vi "_037.vi"() -> ()   [LabVIEW 2024]
panel:
  out "C":dbl
  in  "B":dbl
  in  "A":dbl
  in  "Ring":u16(ring) items=["Add"=10, "Sub"=20, "Mul"=30, "Div"=40]
  out "C":dbl
  in  "B":dbl
  in  "A":dbl
  in  "Enum":enum16{"Add", "Sub", "Mul", "Div"}(ring)
  # "Enum :"
  # "Ring :"
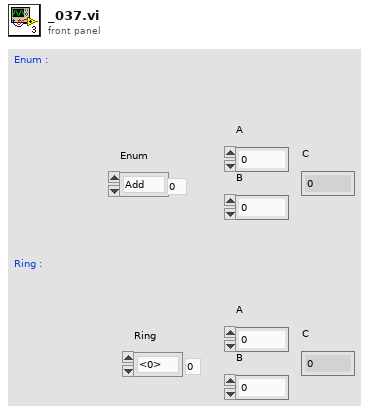
[diagram p1: front panel]
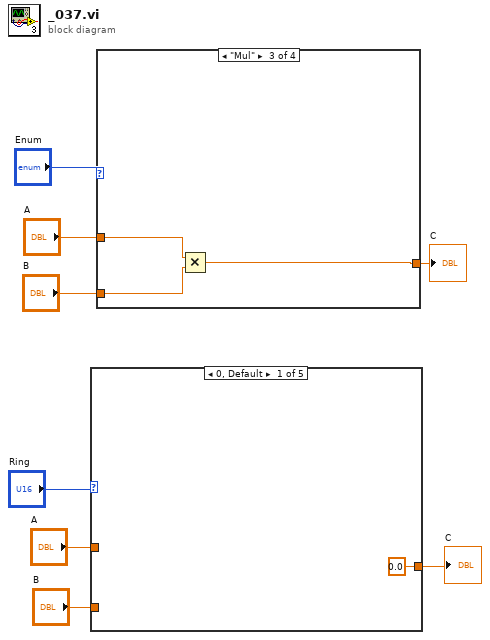
[diagram p0: block diagram]
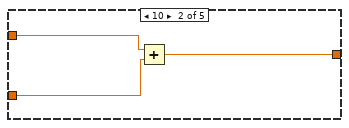
[diagram p2: hidden frame]
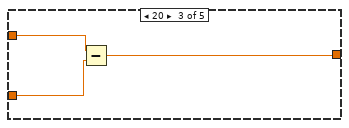
[diagram p3: hidden frame]
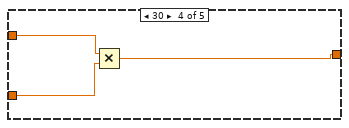
[diagram p4: hidden frame]
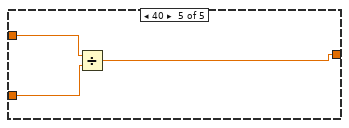
[diagram p5: hidden frame]
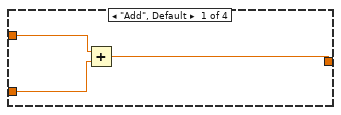
[diagram p6: hidden frame]
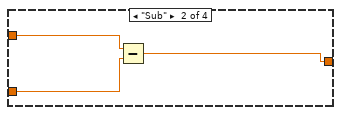
[diagram p7: hidden frame]
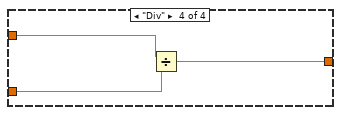
[diagram p8: hidden frame]
diagram:
  n1 = case shown="0, Default" "Ring" {
    tunnel: "A" -> [_ w12 w15 w18 w21]
    tunnel: "B" -> [_ w11 w14 w17 w20]
    tunnel: [0.0 w10 w13 w16 w19] -> w1
    frame 0, Default {
    }
    frame 10 {
      n2 = Add(x=w12, y=w11) -> (x+y=w10:dbl)
    }
    frame 20 {
      n3 = Subtract(x=w15, y=w14) -> (x-y=w13:dbl)
    }
    frame 30 {
      n4 = Multiply(x=w18, y=w17) -> (x*y=w16:dbl)
    }
    frame 40 {
      n5 = Divide(x=w21, y=w20) -> (x/y=w19:dbl)
    }
  }
  "C" <- w1
  n6 = case shown="\"Mul\"" "Enum" {
    tunnel: "A" -> [w24 w27 w30 w33]
    tunnel: "B" -> [w23 w26 w29 w32]
    tunnel: [w22 w25 w28 w31] -> w5
    frame "Add", Default {
      n7 = Add(x=w24, y=w23) -> (x+y=w22:dbl)
    }
    frame "Sub" {
      n8 = Subtract(x=w27, y=w26) -> (x-y=w25:dbl)
    }
    frame "Mul" {
      n9 = Multiply(x=w30, y=w29) -> (x*y=w28:dbl)
    }
    frame "Div" {
      n10 = Divide(x=w33, y=w32) -> (x/y=w31:dbl)
    }
  }
  "C" <- w5
